vi "MainSin.vi"() -> ()   [LabVIEW 2025]
uses:
  StateMachineCTL.ctl
  <vilib>/DAQmx/read.llb/DAQmx Read (Analog 1D Wfm NChan NSamp).vi
  <vilib>/DAQmx/write.llb/DAQmx Write (Analog DBL 1Chan 1Samp).vi
  <vilib>/DAQmx/miscellaneous.llb/DAQmx Fill In Error Info.vi
  <vilib>/ptbypt/NI_PtbyPt.lvlib
panel:
  out "Waveform Chart 2":waveform(dbl)[](graph)
  out "Boolean":bool
  in  "x*y":dbl=5.0 format="%#_13g"
  in  "Exit":bool
  in  "Pause Button":bool
  in  "Media Stop Button":bool
  in  "Play Button":bool
  in  "Amp":dbl(slide) scale=0.0..10.0
  in  "Freq":dbl(knob) scale=0.0..5.0
  out "Waveform Chart":dbl(graph)
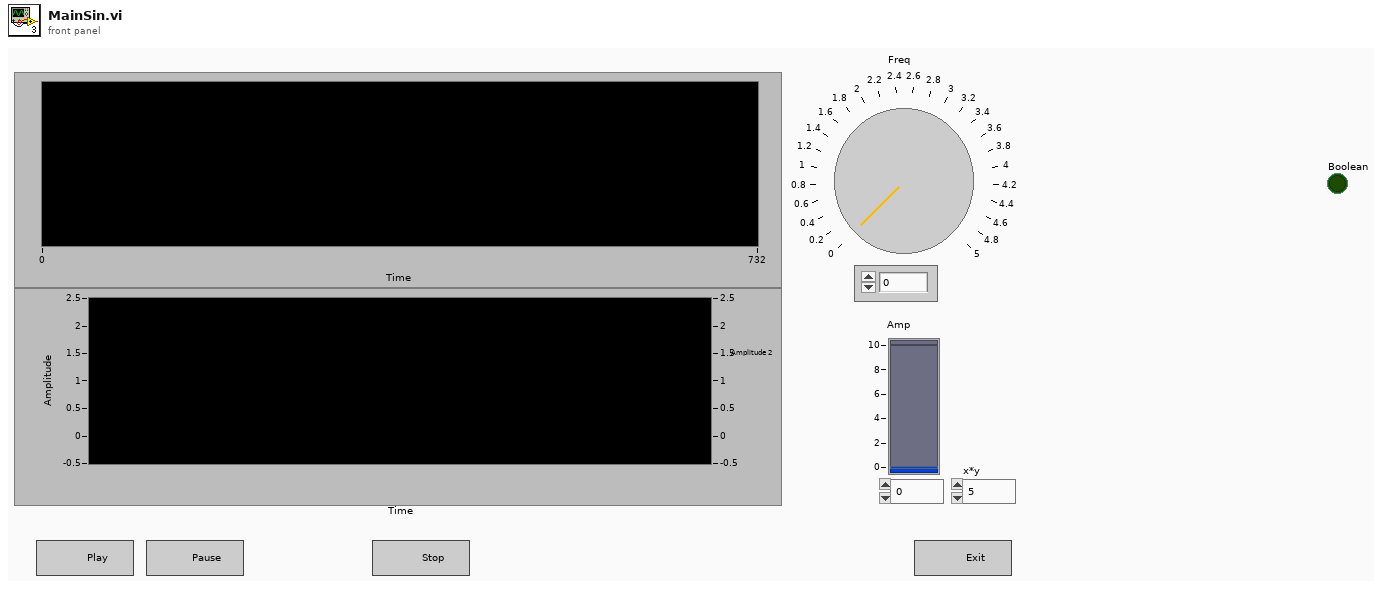
[diagram p1: front panel]
types:
  T1 = typedef "StateMachineCTL.ctl" = enum16{"Ini", "Play", "Pause", "Stop", "Exit"}
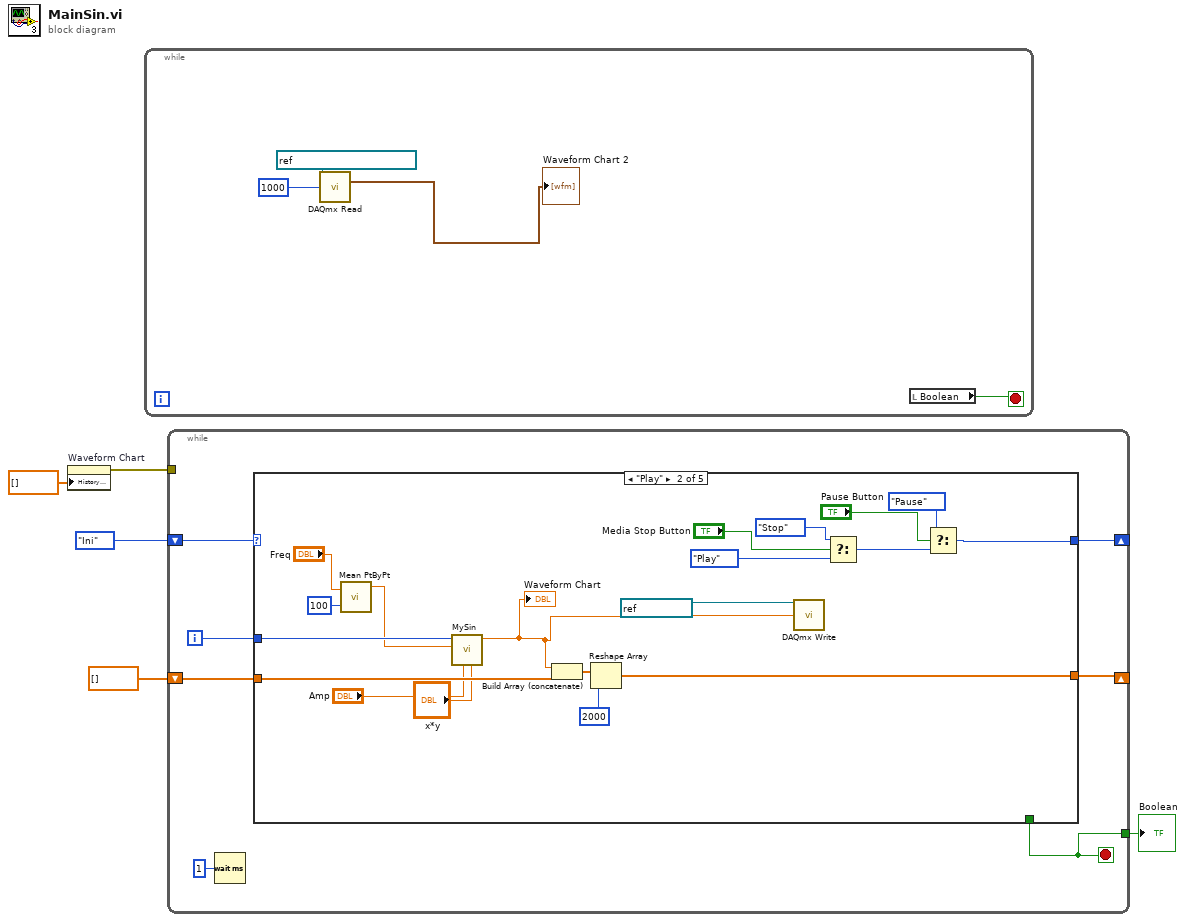
[diagram p0: block diagram]
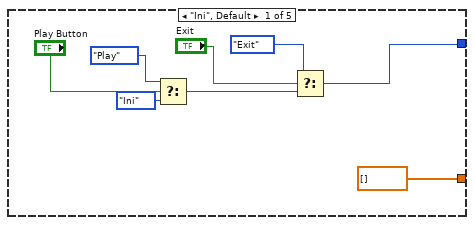
[diagram p2: hidden frame]
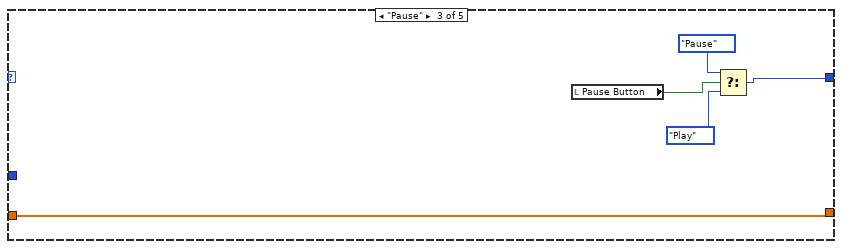
[diagram p3: hidden frame]
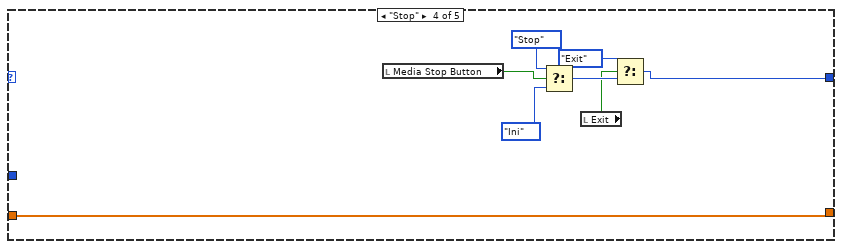
[diagram p4: hidden frame]
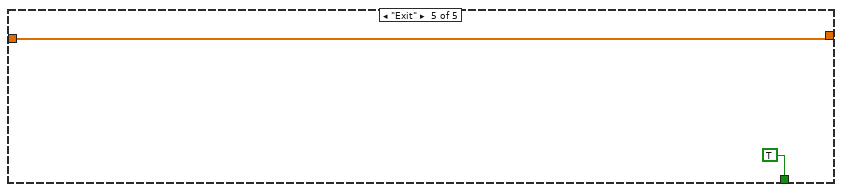
[diagram p5: hidden frame]
diagram:
  n1 = property on="Waveform Chart" class="WFChart (strict)"("History Data"=dbl[] []) -> (error out=w3:errorcluster)  [unwired: 2 in, 1 out]
  n2 = while {
    stop <- w9 stop-if-true
    n3 = call-poly <vilib>:"DAQmx Read.vi"("task/channels in"=refnum<k21> "MyAccelerationLNEC", "number of samples per channel"=1000) -> ("data"=→"Waveform Chart 2":waveform(dbl)[])  [unwired: 11 in, 2 out]
    n4 = local read "Boolean"() -> (w9:bool)
  }
  n5 = while {
    shift-right: [w15] -> _
    shift-left: dbl[] [] -> [w13]
    shift-right: [w12] -> _
    shift-left: StateMachineCTL."Ini" ("Enum") -> [w16]
    tunnel: w3 -> [_]
    tunnel: [w10] -> w1
    i -> [w14]
    stop <- w10 stop-if-true
    n6 = Wait (ms)(milliseconds to wait=u32 1) -> ()  [unwired: 1 out]
    n7 = case shown="\"Play\"" w16 {
      tunnel: [dbl[] [] w28 w44 w53 w58] -> w15
      tunnel: w14 -> [_ w43 _ _ _]
      tunnel: w13 -> [_ w40 w44 w53 w58]
      tunnel: [w17 w32 w46 w49 _] -> w12
      tunnel: [_ _ _ _ TRUE] -> w10
      frame "Ini", Default {
        n8 = Select(t=StateMachineCTL."Play" ("Enum"), s="Play Button", f=StateMachineCTL."Ini") -> (s? t:f=w18:T1)
        n9 = Select(t=StateMachineCTL."Exit" ("Enum"), s="Exit", f=w18) -> (s? t:f=w17:T1)
      }
      frame "Play" {
        n10 = call <vilib>:"Mean PtByPt.vi"("x"="Freq", "sample length"=100) -> ("mean"=w29:dbl)  [unwired: 2 in, 1 out]
        n11 = call "MySin.vi"("x*y"="x*y", "AMP"="Amp", "Freq"=w29, "Numeric 3"=w43) -> ("Numeric 2"=w26:dbl)  [unwired: 6 in, 1 out]
        "Waveform Chart" <- w26
        n12 = Build Array (concatenate)(w26, w40) -> (w41:dbl[])
        n13 = Reshape Array(w41, 2000 ("dimension size")) -> (w28:dbl[])
        n14 = call-poly <vilib>:"DAQmx Write.vi"("task/channels in"=refnum<k21> "sinWave", "data"=w26) -> ()  [unwired: 11 in, 3 out]
        n15 = Select(t=StateMachineCTL."Stop" ("Enum"), s="Media Stop Button", f=StateMachineCTL."Play" ("Enum")) -> (s? t:f=w35:T1)
        n16 = Select(t=StateMachineCTL."Pause", s="Pause Button", f=w35) -> (s? t:f=w32:T1)
      }
      frame "Pause" {
        n17 = local read "Pause Button"() -> (w45:bool)
        n18 = Select(t=StateMachineCTL."Pause", s=w45, f=StateMachineCTL."Play") -> (s? t:f=w46:T1)
      }
      frame "Stop" {
        n19 = local read "Media Stop Button"() -> (w54:bool)
        n20 = Select(t=StateMachineCTL."Stop", s=w54, f=StateMachineCTL."Ini") -> (s? t:f=w52:T1)
        n21 = local read "Exit"() -> (w51:bool)
        n22 = Select(t=StateMachineCTL."Exit", s=w51, f=w52) -> (s? t:f=w49:T1)
      }
      frame "Exit" {
      }
    }
  }
  "Boolean" <- w1
